vi "Convert PNG to VIs.vi"(8 "error in (no error)":errorcluster, 11 "selected path":path) -> (0 "error out":errorcluster, 3 "directory copy":path)   [LabVIEW 2015]
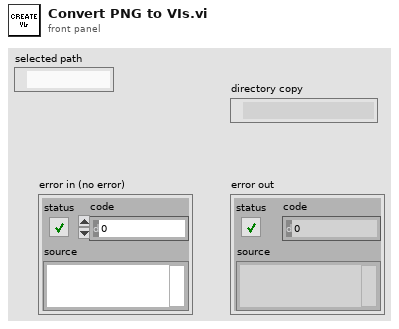
[diagram p1: front panel]
types:
  T1 = cluster{"left":i16, "top":i16, "right":i16, "bottom":i16}
  T2 = typedef "imagedata.ctl" = cluster{"image type":i32, "image depth":i32, "image":u8[], "mask":u8[], "colors":u32[], "Rectangle":cluster{"left":i16, "top":i16, "right":i16, "bottom":i16}}
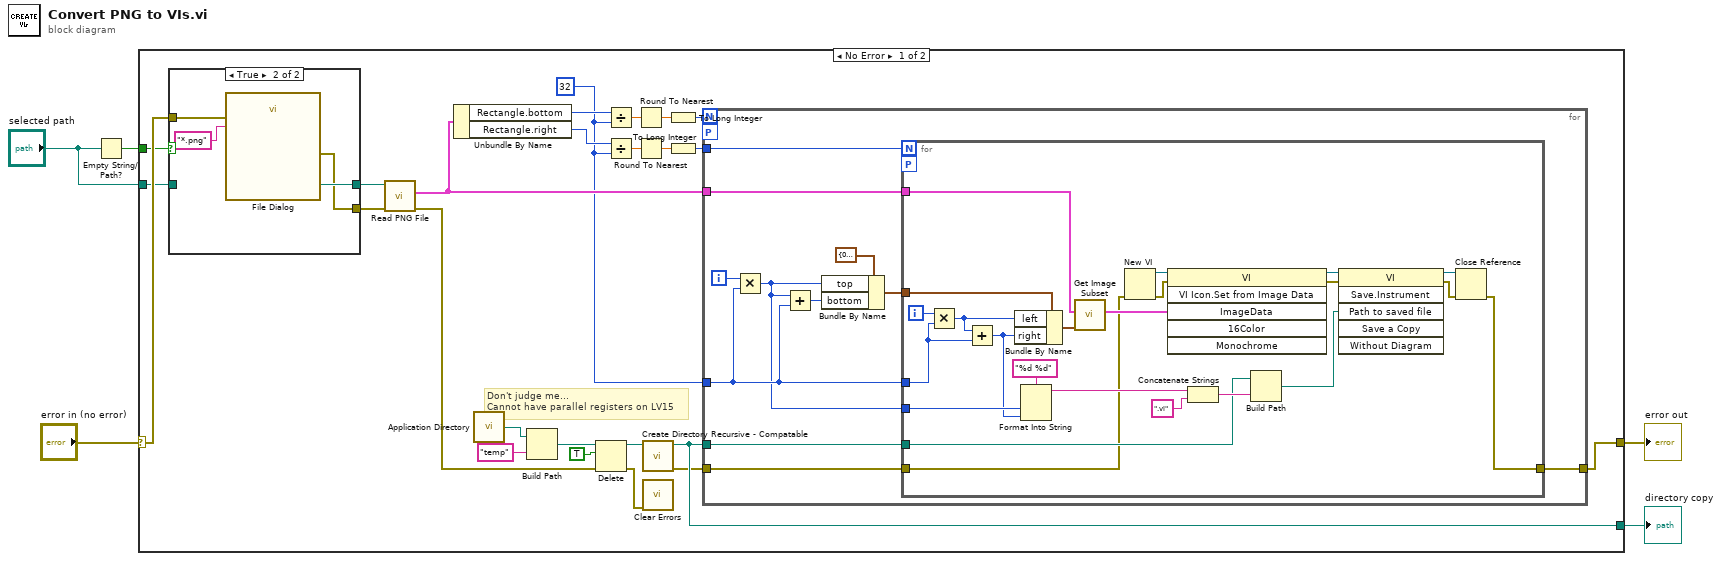
[diagram p0: block diagram]
diagram:
  n1 = Empty String/Path?(string/path="selected path") -> (empty?=w2:bool)
  n2 = case shown="No Error" "error in (no error)" {
    selector: "error in (no error)" -> [w13 w71]
    tunnel: [w10 _] -> w5
    tunnel: [w12 w71] -> w3
    tunnel: w2 -> [w7 _]
    tunnel: "selected path" -> [w6 _]
    frame No Error {
      w19 = i16 32 ("y")
      # "Don't judge me...\nCannot have parallel registers on LV15"
      n3 = case shown="True" w7 {
        tunnel: [w32 w36] -> w25
        tunnel: [w31 w34] -> w15
        tunnel: w13 -> [w31 w33]
        tunnel: w6 -> [w32 _]
        frame False {
        }
        frame True {
          n4 = call "File Dialog"("error in"=w33, "pattern (all files)"="*.png") -> ("selected path"=w36:path, "error out"=w34:errorcluster)  [unwired: 10 in, 2 out]
        }
      }
      n5 = call <vilib>:"Read PNG File.vi"("error in (no error)"=w15, "path to PNG file"=w25) -> ("error out"=w14:errorcluster, "image data"=w30:T2)  [unwired: 7 in, 1 out]
      n6 = Unbundle By Name(w30) -> ("Rectangle.bottom"=w29:i16, "Rectangle.right"=w20:i16)
      n7 = call <vilib>:"Application Directory.vi"() -> ("Application Directory"=w23:path)
      n8 = Build Path(base path=w23, name or relative path="temp") -> (appended path=w24:path)
      n9 = Delete(path (use dialog)=w24, entire hierarchy (F)=TRUE, error in=w14) -> (deleted path=w11:path, error out=w8:errorcluster)  [unwired: 2 in, 1 out]
      n10 = Divide(x=w29, y=w19) -> (x/y=w27:dbl)
      n11 = Divide(x=w20, y=w19) -> (x/y=w28:dbl)
      n12 = Round To Nearest(number=w27) -> (nearest integer value=w18:dbl)
      n13 = Round To Nearest(number=w28) -> (nearest integer value=w26:dbl)
      n14 = call <resource>:"Create Directory Recursive - Compatable.vi"("directory"=w11) -> ("error out"=w9:errorcluster, "directory copy"=w10:path)  [unwired: 8 in, 1 out]
      n15 = call <vilib>:"Clear Errors.vi"("error in (no error)"=w8) -> ()  [unwired: 5 in, 2 out]
      n16 = To Long Integer(number=w18) -> (32bit integer=w17:i32)
      n17 = To Long Integer(number=w26) -> (32bit integer=w16:i32)
      n18 = for {
        N: w17 -> [_]
        tunnel: w30 -> [w47]
        tunnel: w16 -> [w46]
        tunnel: w19 -> [w43]
        tunnel: w10 -> [w40]
        workers-P: _ -> [_]
        tunnel: w9 -> [w38]
        tunnel: [w37] -> w12
        i -> [w44]
        n19 = Multiply(x=w44, y=w43) -> (x*y=w41:i32)
        n20 = Add(x=w41, y=w43) -> (x+y=w42:i32)
        n21 = Bundle By Name(cluster=T1 {"left"=0, "top"=0, "right"=0, "bottom"=0} ("subset rect"), "top"=w41, "bottom"=w42) -> (w45:T1)
        n22 = for {
          N: w46 -> [_]
          tunnel: w45 -> [w70]
          tunnel: w47 -> [w69]
          tunnel: w43 -> [w67]
          tunnel: w41 -> [w54]
          tunnel: w40 -> [w51]
          workers-P: _ -> [_]
          tunnel: w38 -> [w50]
          tunnel: [w48] -> w37
          i -> [w68]
          n23 = Multiply(x=w68, y=w67) -> (x*y=w53:i32)
          n24 = Add(x=w53, y=w67) -> (x+y=w52:i32)
          n25 = Bundle By Name(cluster=w70, "left"=w53, "right"=w52) -> (w57:T1)
          n26 = Format Into String(format string="%d %d", w54, w52) -> (resulting string=w55:string)  [unwired: 2 in, 1 out]
          n27 = call <vilib>:"Get Image Subset.vi"("subset rect"=w57, "image data"=w69) -> ("image subset"=w65:T2)  [unwired: 4 in, 1 out]
          n28 = New VI(8:w50) -> (0:w49:errorcluster, 3:w66:refnum<vi>)  [unwired: 6 in]
          n29 = invoke class="VI" method="VI Icon.Set from Image Data"(reference=w66, error in=w49, "ImageData"=w65) -> (reference out=w64:refnum<vi>, error out=w60:errorcluster)  [unwired: 3 in, 4 out]
          n30 = Concatenate Strings(w55, ".vi" ("string")) -> (w63:string)
          n31 = Build Path(base path=w51, name or relative path=w63) -> (appended path=w61:path)
          n32 = invoke class="VI" method="Save.Instrument"(reference=w64, error in=w60, "Path to saved file"=w61) -> (reference out=w59:refnum<vi>, error out=w58:errorcluster)  [unwired: 3 in, 4 out]
          n33 = Close Reference(reference=w59, error in (no error)=w58) -> (error out=w48:errorcluster)
        }
      }
    }
    frame Error {
    }
  }
  "error out" <- w3
  "directory copy" <- w5
